vi "fakespectra2.vi"(0 "LT preset":dbl) -> (1 "Waveform Graph":u32[](graph), 2 "LT out":dbl, 3 "RT out":dbl)   [LabVIEW 2015]
uses:
  <vilib>/Utility/file.llb/Read From Spreadsheet File (DBL).vi
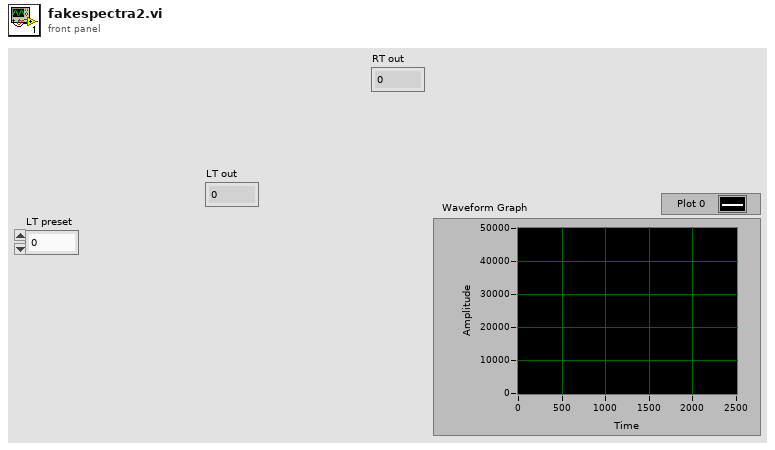
[diagram p1: front panel]
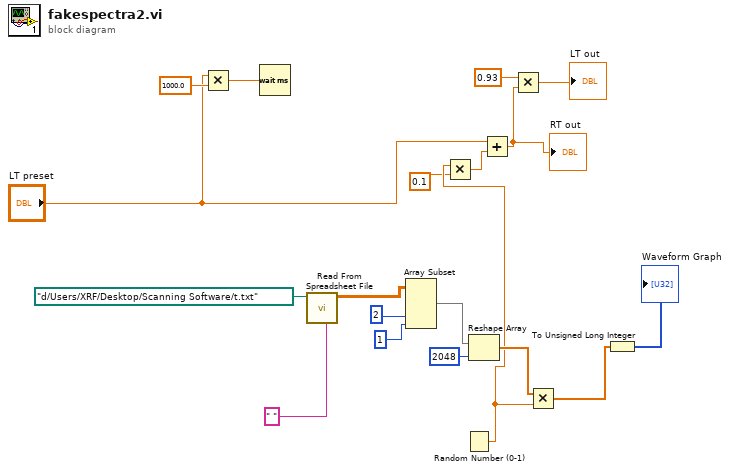
[diagram p0: block diagram]
diagram:
  n1 = Multiply(x="LT preset", y=1000.0) -> (x*y=w4:dbl)
  n2 = Wait (ms)(milliseconds to wait=w4) -> ()  [unwired: 1 out]
  n3 = call-poly <vilib>:"Read From Spreadsheet File.vi"("delimiter (\\t)"=" ", "file path (dialog if empty)"=path "d:/Users/XRF/Desktop/Scanning Software/t.txt") -> ("all rows"=w17:dbl[][])  [unwired: 5 in, 4 out]
  n4 = Array Subset(array=w17, index (col)=2 ("index"), length (col)=1 ("length")) -> (w14:dbl[][])  [unwired: 2 in]
  n5 = Random Number (0-1)() -> (number: 0 to 1=w9:dbl)
  n6 = Multiply(x=w9, y=0.1) -> (x*y=w7:dbl)
  n7 = Reshape Array(w14, 2048 ("dimension size")) -> (w11:dbl[])
  n8 = Add(x="LT preset", y=w7) -> (x+y=w2:dbl)
  "RT out" <- w2
  n9 = Multiply(x=0.93, y=w2) -> (x*y=→"LT out":dbl)
  n10 = Multiply(x=w11, y=w9) -> (x*y=w10:dbl[])
  n11 = To Unsigned Long Integer(number=w10) -> (unsigned 32bit integer=→"Waveform Graph":u32[])
